vi "AlazarReadU16.vi"(0 "Handle":u64, 1 "Channel":u32(ring)=1 items=["A"=1, "B"=2, "C"=4, "D"=8], 2 "Record":i32, 3 "Transfer Offset":i32, 4 "Transfer Length":u32, 5 "error in (no error)":errorcluster) -> (14 "Handle":u64, 15 "Buffer":u16[](array[numeric]), 18 "Return Code":u32, 19 "error out":errorcluster)   [LabVIEW 2018]
doc: "Read all or part of a record from an acquisition to on-board memory from on-board memory to a buffer in host memory. The record must be less than 2,147,483,648 samples long."
uses:
  ATSApi.dll
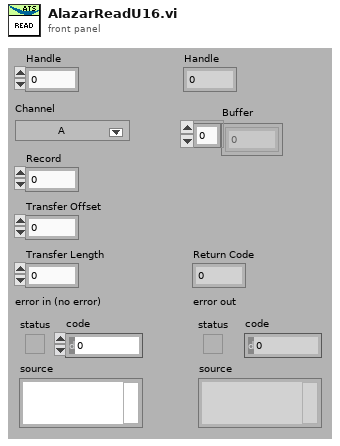
[diagram p1: front panel]
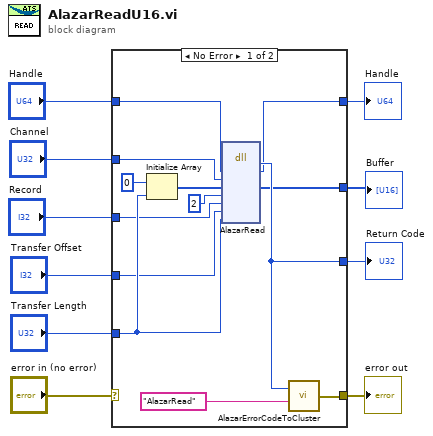
[diagram p0: block diagram]
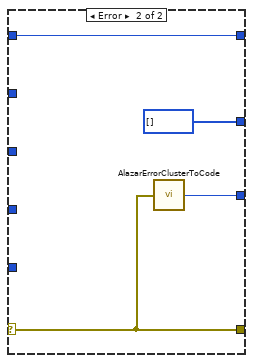
[diagram p2: hidden frame]
diagram:
  n1 = case shown="No Error" "error in (no error)" {
    selector: "error in (no error)" -> [_ w27]
    tunnel: [w20 w27] -> w9
    tunnel: [w22 w26] -> w8
    tunnel: "Handle" -> [w23 w25]
    tunnel: [w19 w25] -> w6
    tunnel: "Transfer Length" -> [w17 _]
    tunnel: "Transfer Offset" -> [w16 _]
    tunnel: "Record" -> [w15 _]
    tunnel: "Channel" -> [w12 _]
    tunnel: [w11 u16[] []] -> w1
    frame No Error {
      n2 = Initialize Array(u16 0, w17) -> (w14:u16[])
      n3 = dll-call lib="ATSApi.dll" fn="AlazarRead"("handle"=w23, "channelId"=w12, "buffer"=w14, "elementSize"=2, "record"=w15, "transferOffset"=w16, "transferLength"=w17) -> ("return type"=w22:u32, "handle"=w19:u64, "buffer"=w11:u16[])  [unwired: 8 in, 2 out]
      n4 = call "AlazarErrorCodeToCluster.vi"("Message"="AlazarRead", "Error Code"=w22) -> ("error out"=w20:errorcluster)
    }
    frame Error {
      n5 = call "AlazarErrorClusterToCode.vi"("error in (no error)"=w27) -> ("Error Code"=w26:u32)
    }
  }
  "Handle" <- w6
  "error out" <- w9
  "Return Code" <- w8
  "Buffer" <- w1
